vi "Save_Data.vi"(9 "Path":path=path "C:/Documents and Settings/en51tf/Desktop/trash/test.xls  ", 10 "appended array":T1[](array[typedef])) -> ()   [LabVIEW 2011]
uses:
  Controls/XY_Plot_Cluster.ctl
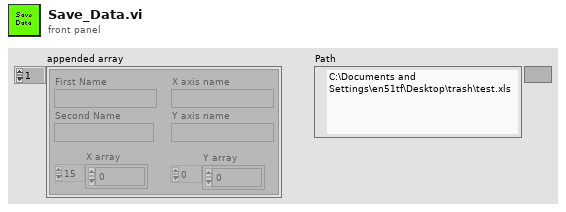
[diagram p1: front panel]
types:
  T1 = typedef "XY_Plot_Cluster.ctl" = cluster{"First Name":string, "Second Name":string, "X axis name":string, "Y axis name":string, "X array":dbl[], "Y array":dbl[]}
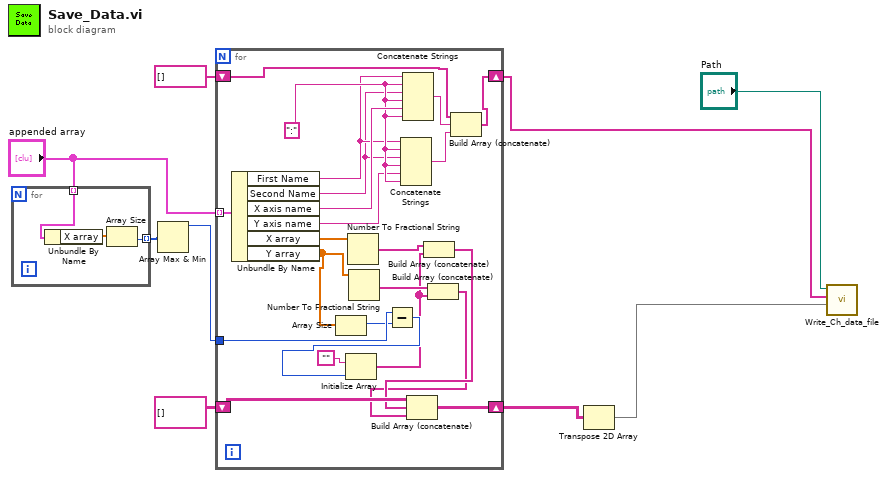
[diagram p0: block diagram]
diagram:
  n1 = for {
    tunnel: "appended array" -> [w12] mode=indexing
    tunnel: [w10] -> w4 mode=indexing
    n2 = Unbundle By Name(w12) -> ("X array"=w11:dbl[])
    n3 = Array Size(array=w11) -> (size(s)=w10:i32)
  }
  n4 = Array Max & Min(array=w4) -> (max value=w3:i32)  [unwired: 3 out]
  n5 = for {
    shift-right: [w34] -> w1
    shift-left: string[][] [] -> [w35]
    tunnel: "appended array" -> [w33] mode=indexing
    shift-right: [w24] -> w7
    shift-left: string[] [] -> [w25]
    tunnel: w3 -> [w20]
    w31 = ":" ("string")
    n6 = Unbundle By Name(w33) -> ("First Name"=w30:string, "Second Name"=w29:string, "X axis name"=w32:string, "Y axis name"=w28:string, "X array"=w23:dbl[], "Y array"=w22:dbl[])
    n7 = Array Size(array=w22) -> (size(s)=w19:i32)
    n8 = Number To Fractional String(number=w23) -> (F-format string=w18:string[])  [unwired: 1 in, 2 out]
    n9 = Number To Fractional String(number=w22) -> (F-format string=w16:string[])  [unwired: 1 in, 2 out]
    n10 = Subtract(x=w20, y=w19) -> (x-y=w17:i32)
    n11 = Initialize Array("", w17) -> (w15:string[])
    n12 = Concatenate Strings(w30, w31, w29, w31, w28, w31) -> (w27:string)
    n13 = Concatenate Strings(w30, w31, w29, w31, w32, w31) -> (w26:string)
    n14 = Build Array (concatenate)(w18, w15) -> (w14:string[])
    n15 = Build Array (concatenate)(w16, w15) -> (w13:string[])
    n16 = Build Array (concatenate)(w35, w14, w13) -> (w34:string[][])
    n17 = Build Array (concatenate)(w25, w26, w27) -> (w24:string[])
  }
  n18 = Transpose 2D Array(2D array=w1) -> (transposed array=w6:string[][])
  n19 = call "Write_Ch_data_file.vi"("Channel Values"=w6, "Channel names"=w7, "Filename"="Path") -> ()  [unwired: 5 in, 4 out]
